vi "camera shutter.vi"(11 "Camera Input Switch":bool[](array[boolean])) -> (3 "Camera Output Switch":bool[](array[boolean]))   [LabVIEW 2014]
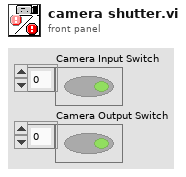
[diagram p1: front panel]
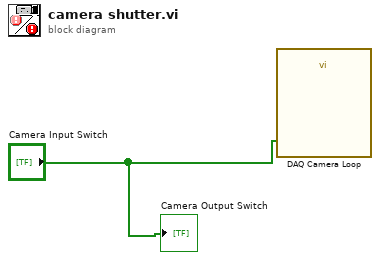
[diagram p0: block diagram]
diagram:
  n1 = call "DAQ Camera Loop"("data"="Camera Input Switch") -> ()  [unwired: 17 in, 2 out]
  "Camera Output Switch" <- "Camera Input Switch"
